vi "Stop.vi"(8 "error in (no error)":errorcluster caption="entrée d'erreur (pas d'erreur)", 11 "Process (Default) en entrée":refnum<class "Process (Default).lvclass">) -> (0 "error out":errorcluster caption="sortie d'erreur", 3 "Process (Default) en sortie":refnum<class "Process (Default).lvclass">)   [LabVIEW 2020, in "Library Instrument & Equipement.lvlib" / "Process (Default).lvclass"]
uses:
  Process (Default).lvclass
  Process (Default).lvclass/Process (Default).ctl
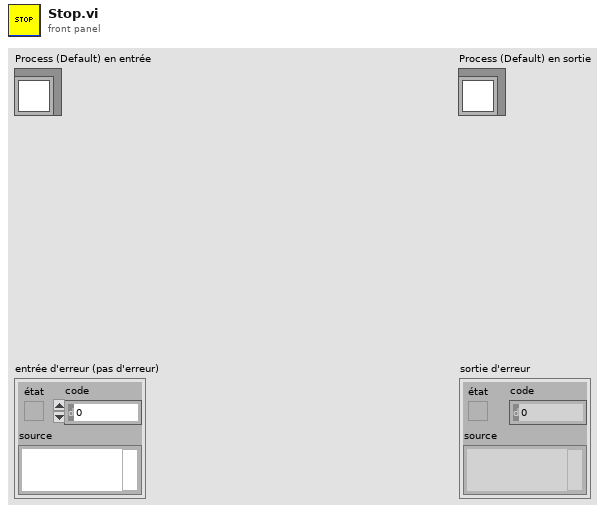
[diagram p1: front panel]
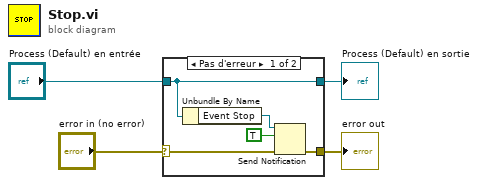
[diagram p0: block diagram]
diagram:
  n1 = case shown="Pas d'erreur" "error in (no error)" {
    selector: "error in (no error)" -> [w9 w11]
    tunnel: [w8 w11] -> w3
    tunnel: [w7 w10] -> w1
    tunnel: "Process (Default) en entrée" -> [w7 w10]
    frame No Error {
      n2 = Unbundle By Name(w7) -> ("Event Stop"=w6:refnum<notifier>)
      n3 = Send Notification(notification=TRUE, notifier=w6, error in (no error)=w9) -> (error out=w8:errorcluster)  [unwired: 1 out]
    }
    frame Error {
    }
  }
  "error out" <- w3
  "Process (Default) en sortie" <- w1
